vi "LaserEnable.vi"(4 "Enable":bool, 5 "COM Port":refnum<visa-resource-name>="COM6") -> ()   [LabVIEW 2020]
uses:
  <vilib>/Instr/_visa.llb/VISA Configure Serial Port (Instr).vi
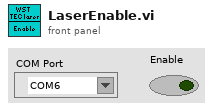
[diagram p1: front panel]
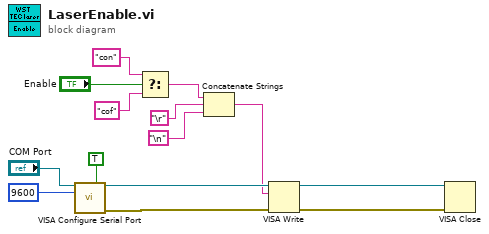
[diagram p0: block diagram]
diagram:
  n1 = call-poly "VISA Configure Serial Port"("VISA resource name"="COM Port", "Enable Termination\nChar (T)"=TRUE ("Enable Termination\nChar (T)"), "baud rate (9600)"=u32 9600) -> ("VISA resource name out"=w11:refnum<visa-resource-name>, "error out"=w10:errorcluster)  [unwired: 11 in]
  n2 = Select(t="con", s="Enable", f="cof") -> (s? t:f=w4:string)
  n3 = Concatenate Strings(w4, "\r", "\n") -> (w1:string)
  n4 = VISA Write(VISA resource name=w11, write buffer=w1, error in (no error)=w10) -> (VISA resource name out=w9:refnum<visa-resource-name>, error out=w8:errorcluster)  [unwired: 1 out]
  n5 = VISA Close(VISA resource name=w9, error in (no error)=w8) -> ()  [unwired: 1 out]
